vi "Pendulum connect.vi"(10 "latency_mS":u8, 11 "instance":i32) -> (3 "function return":i32)   [LabVIEW 2025, in "pendulumApp.lvlib"]
doc: "OOTB_API int Pendulum_connect(int instance, unsigned char latency_mS);"
uses:
  pendulumApp.lvlib
  pendulumApp.dll
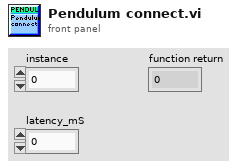
[diagram p1: front panel]
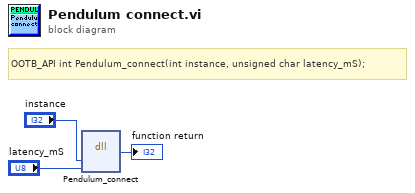
[diagram p0: block diagram]
diagram:
  # "OOTB_API\tint Pendulum_connect(int instance, unsigned char latency_mS);"
  n1 = dll-call lib="C:/Users/noaht/School/Fall 2025/Controls Lab/Lab 3/FA25_pend_Lab3_4/SADI_Pendulum_lib/pendulumApp.*" fn="Pendulum_connect"("instance"="instance", "latency_mS"="latency_mS") -> (→"function return":i32)  [unwired: 5 in, 2 out]
